vi "Butterfly_extract_VPI_VRL - PolyMorphic.vi"   [LabVIEW 2013]
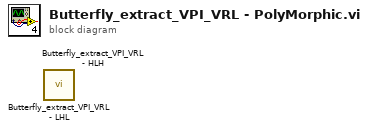
[diagram p0: block diagram]
diagram:
  n1 = call "Butterfly_extract_VPI_VRL - LHL.vi"() -> ()  [unwired: 10 in, 2 out]
  n2 = call "Butterfly_extract_VPI_VRL - HLH.vi"() -> ()  [unwired: 10 in, 2 out]
